vi "HandlePass.vi"(8 "error in (no error)":errorcluster, 10 "Perform?":bool, 11 "DoubleClick?":bool) -> (0 "error out":errorcluster, 1 "Call?":bool, 2 "PassState":T2, 3 "PassType":T1)   [LabVIEW 2013]
doc: "Determines which pass to perform, their state, and whether to actually call the pass VI.\n\nThe ground pass is activated with a single click (<B>DoubleClick?</B> = F), and reset with a single click.\nThe elevated pass is activated with a double click (<B>DoubleClick</B> = T) and reset with a double click."
uses:
  PassState.ctl
  PassType.ctl
  HandlePassAction.ctl
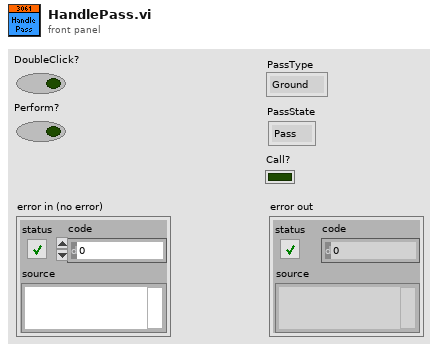
[diagram p1: front panel]
types:
  T1 = typedef "PassType.ctl" = enum16{"Ground", "Elevated"}
  T2 = typedef "PassState.ctl" = enum16{"Pass", "Stop"}
  T3 = typedef "HandlePassAction.ctl" = enum16{"Idle", "Ground", "Elevated"}
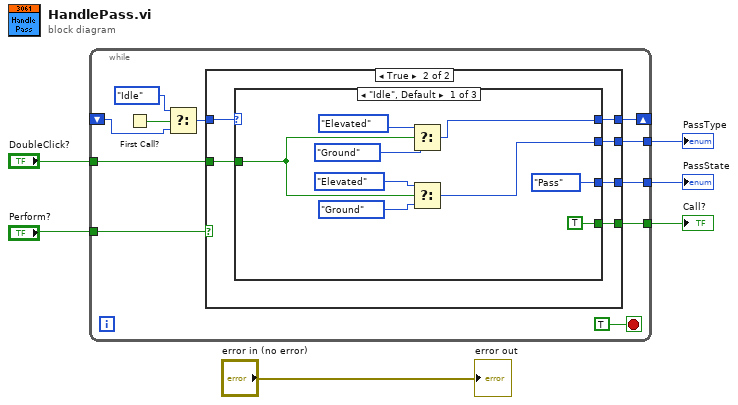
[diagram p0: block diagram]
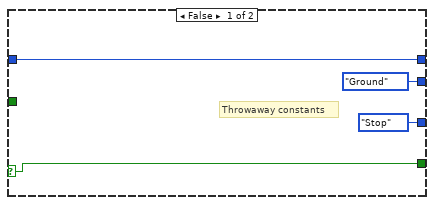
[diagram p2: hidden frame]
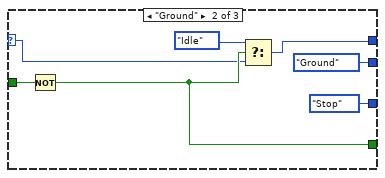
[diagram p3: hidden frame]
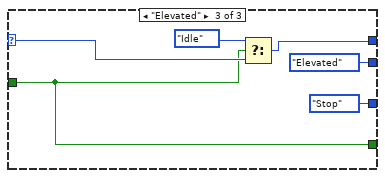
[diagram p4: hidden frame]
diagram:
  n1 = while {
    tunnel: "Perform?" -> [w16]
    shift-right: [w15] -> _
    shift-left: _ -> [w12]
    tunnel: "DoubleClick?" -> [w10]
    tunnel: [w9] -> w4
    tunnel: [w8] -> w3
    tunnel: [w7] -> w2
    stop <- TRUE stop-if-true
    n2 = First Call?() -> (First Call?: T/F=w13:bool)
    n3 = Select(t=HandlePassAction."Idle", s=w13, f=w12) -> (s? t:f=w11:T3)
    n4 = case shown="True" w16 {
      selector: w16 -> [w20 _]
      tunnel: w11 -> [w21 w27]
      tunnel: [w21 w25] -> w15
      tunnel: w10 -> [_ w26]
      tunnel: [PassType."Ground" ("PassType") w24] -> w9
      tunnel: [PassState."Stop" ("PassState") w23] -> w8
      tunnel: [w20 w22] -> w7
      frame False {
        # "Throwaway constants"
      }
      frame True {
        n5 = case shown="\"Idle\", Default" w27 {
          selector: w27 -> [_ w37 w46]
          tunnel: w26 -> [w30 w41 w45]
          tunnel: [w36 w39 w44] -> w25
          tunnel: [w31 PassType."Ground" ("PassType") PassType."Elevated" ("PassType")] -> w24
          tunnel: [PassState."Pass" ("PassState") PassState."Stop" ("PassState") PassState."Stop" ("PassState")] -> w23
          tunnel: [TRUE w38 w45] -> w22
          frame "Idle", Default {
            n6 = Select(t=HandlePassAction."Elevated", s=w30, f=HandlePassAction."Ground") -> (s? t:f=w36:T3)
            n7 = Select(t=PassType."Elevated" ("PassType"), s=w30, f=PassType."Ground" ("PassType")) -> (s? t:f=w31:T1)
          }
          frame "Ground" {
            n8 = Not(x=w41) -> (.not. x?=w38:bool)
            n9 = Select(t=HandlePassAction."Idle", s=w38, f=w37) -> (s? t:f=w39:T3)
          }
          frame "Elevated" {
            n10 = Select(t=HandlePassAction."Idle", s=w45, f=w46) -> (s? t:f=w44:T3)
          }
        }
      }
    }
  }
  "PassState" <- w3
  "PassType" <- w4
  "Call?" <- w2
  "error out" <- "error in (no error)"
